vi "VMC-4.vi"(11 "数组":u8[](array[numeric])) -> (0 "侧向过载":i16, 1 "航向角速率":i16, 2 "当地纬度数据输入":i16, 3 "滚转角速率":i16, 4 "轴向过载":i16, 5 "俯仰角速率":i16, 6 "法向过载":i16, 7 "当地重力加速度":i16)   [LabVIEW 2012]
uses:
  index-i16.vi
  XX-I16.vi
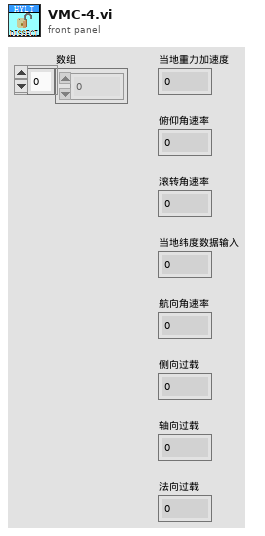
[diagram p1: front panel]
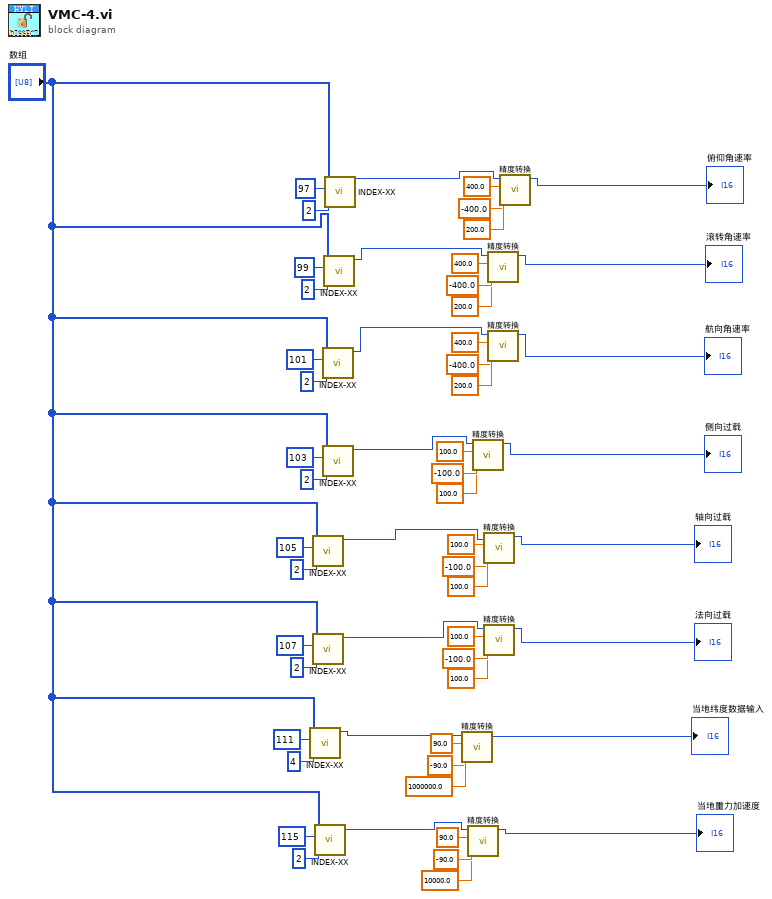
[diagram p0: block diagram]
diagram:
  n1 = call-poly "INDEX-XX.vi"("长度"=4, "索引"=111, "数组"="数组") -> ("数值输出"=w16:i16)  [unwired: 8 in]
  n2 = call-poly "INDEX-XX.vi"("长度"=2, "索引"=105, "数组"="数组") -> ("数值输出"=w50:i16)  [unwired: 8 in]
  n3 = call-poly "INDEX-XX.vi"("长度"=2, "索引"=107, "数组"="数组") -> ("数值输出"=w55:i16)  [unwired: 8 in]
  n4 = call-poly "INDEX-XX.vi"("长度"=2, "索引"=115, "数组"="数组") -> ("数值输出"=w25:i16)  [unwired: 8 in]
  n5 = call-poly "INDEX-XX.vi"("长度"=2, "索引"=101, "数组"="数组") -> ("数值输出"=w40:i16)  [unwired: 8 in]
  n6 = call-poly "INDEX-XX.vi"("长度"=2, "索引"=103, "数组"="数组") -> ("数值输出"=w45:i16)  [unwired: 8 in]
  n7 = call-poly "INDEX-XX.vi"("长度"=2, "索引"=99, "数组"="数组") -> ("数值输出"=w35:i16)  [unwired: 8 in]
  n8 = call-poly "INDEX-XX.vi"("长度"=2, "索引"=97, "数组"="数组") -> ("数值输出"=w30:i16)  [unwired: 8 in]
  n9 = call-poly "精度转换.vi"("单位"=1000000.0, "下限"=-90.0, "上限"=90.0, "数值输入"=w16) -> ("输出"=→"当地纬度数据输入":i16)  [unwired: 7 in]
  n10 = call-poly "精度转换.vi"("单位"=10000.0, "下限"=-90.0, "上限"=90.0, "数值输入"=w25) -> ("输出"=→"当地重力加速度":i16)  [unwired: 7 in]
  n11 = call-poly "精度转换.vi"("单位"=100.0, "下限"=-100.0, "上限"=100.0, "数值输入"=w45) -> ("输出"=→"侧向过载":i16)  [unwired: 7 in]
  n12 = call-poly "精度转换.vi"("单位"=100.0, "下限"=-100.0, "上限"=100.0, "数值输入"=w50) -> ("输出"=→"轴向过载":i16)  [unwired: 7 in]
  n13 = call-poly "精度转换.vi"("单位"=100.0, "下限"=-100.0, "上限"=100.0, "数值输入"=w55) -> ("输出"=→"法向过载":i16)  [unwired: 7 in]
  n14 = call-poly "精度转换.vi"("单位"=200.0, "下限"=-400.0, "上限"=400.0, "数值输入"=w35) -> ("输出"=→"滚转角速率":i16)  [unwired: 7 in]
  n15 = call-poly "精度转换.vi"("单位"=200.0, "下限"=-400.0, "上限"=400.0, "数值输入"=w40) -> ("输出"=→"航向角速率":i16)  [unwired: 7 in]
  n16 = call-poly "精度转换.vi"("单位"=200.0, "下限"=-400.0, "上限"=400.0, "数值输入"=w30) -> ("输出"=→"俯仰角速率":i16)  [unwired: 7 in]
